vi "Event handler-VidRec enable.vi"(11 "Enable Video Recording.NewVal":bool) -> ()   [LabVIEW 2013]
uses:
  Typedefs/Read Write Enum.ctl
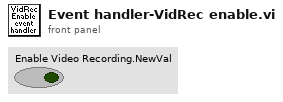
[diagram p1: front panel]
types:
  T1 = typedef "Read Write Enum.ctl" = enum16{"Read", "Write"}
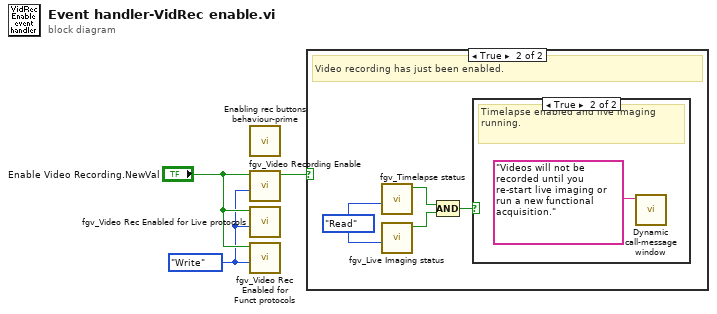
[diagram p0: block diagram]
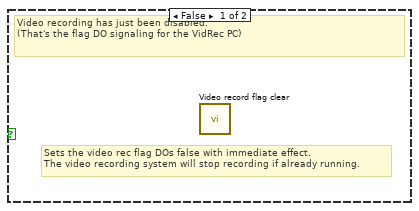
[diagram p2: hidden frame]
diagram:
  w2 = Read_Write_Enum."Write" ("Function")
  n1 = call "Enabling rec buttons behaviour-prime.vi"() -> ()  [unwired: 12 in]
  n2 = call "fgv_Video Recording Enable.vi"("Function"=w2, "Video Recording Enabled"="Enable Video Recording.NewVal") -> ("Video Recording Enabled"=w1:bool)  [unwired: 9 in]
  n3 = call "fgv_Video Rec Enabled for Live protocols.vi"("Function"=w2, "Video Recording Enabled for Live protocols"="Enable Video Recording.NewVal") -> ()  [unwired: 9 in, 1 out]
  n4 = call "fgv_Video Rec Enabled for Funct protocols.vi"("Function"=w2, "Video Recording Enabled for functional acq protocols"="Enable Video Recording.NewVal") -> ()  [unwired: 9 in, 1 out]
  n5 = case shown="True" w1 {
    frame False {
      # "Sets the video rec flag DOs false with immediate effect.\nThe video recording system will stop recording if already running."
      # "Video recording has just been disabled.\n(That's the flag DO signaling for the VidRec PC)"
      n6 = call "Video record flag clear.vi"() -> ()  [unwired: 12 in]
    }
    frame True {
      w7 = Read_Write_Enum."Read" ("Function")
      # "Video recording has just been enabled."
      n7 = call "fgv_Timelapse status.vi"("Function"=w7) -> ("Timelapse?"=w6:bool)  [unwired: 10 in]
      n8 = call "fgv_Live Imaging status.vi"("Function"=w7) -> ("Live Imaging?"=w5:bool)  [unwired: 9 in, 1 out]
      n9 = Compound Arithmetic op=AND(w6, w5) -> (w4:bool)
      n10 = case shown="True" w4 {
        frame False {
        }
        frame True {
          # "Timelapse enabled and live imaging running."
          n11 = call "Dynamic call-message window.vi"("Message"="Videos will not be recorded until you re-start live imaging or run a new functional acquisition." ("message")) -> ()  [unwired: 10 in, 1 out]
        }
      }
    }
  }
